vi "BuildPageArray.vi"(8 "error in (no error)":errorcluster, 10 "Config File Path":path) -> (0 "error out":errorcluster, 2 "Num Pages":i32, 3 "Array":refnum<class "Slide.lvclass">[](array[class]))   [LabVIEW 2017]
uses:
  Slide/Slide.lvclass
  Slide/SlideType.ctl
  <vilib>/regexp/Match Regular Expression.xnode
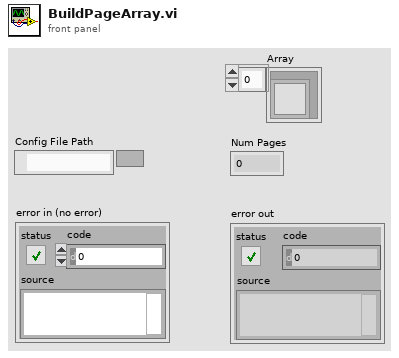
[diagram p1: front panel]
types:
  T1 = typedef "Slide.lvclass/SlideType.ctl" = enum16{"Image", "FP", "BD"}
  T2 = cluster{i32, "BD Slide":refnum<class "Slide.lvclass">}
  T3 = cluster{i32, "BD Slide":refnum<class "Slide.lvclass">}[]
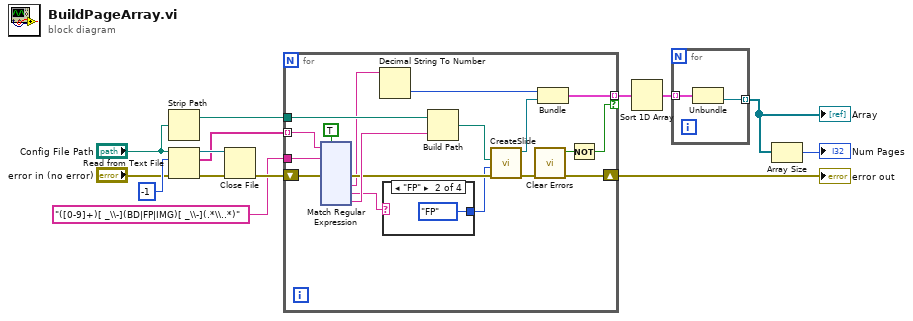
[diagram p0: block diagram]
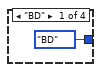
[diagram p2: hidden frame]
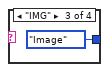
[diagram p3: hidden frame]
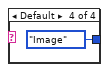
[diagram p4: hidden frame]
diagram:
  n1 = Strip Path(path="Config File Path") -> (stripped path=w6:path)  [unwired: 1 out]
  n2 = Read from Text File(file (use dialog)="Config File Path", count=-1, error in="error in (no error)") -> (refnum out=w11:refnum<file>, text=w10:string[], error out=w12:errorcluster)  [unwired: 1 in, 1 out]
  n3 = Close File(refnum=w11, error in=w12) -> (error out=w9:errorcluster)  [unwired: 1 out]
  n4 = for {
    tunnel: w10 -> [w31] mode=indexing
    shift-right: [w17] -> w4
    shift-left: w9 -> [w29]
    tunnel: "([0-9]+)[ _\\-](BD|FP|IMG)[ _\\-](.*\\..*)" -> [w28]
    tunnel: w6 -> [w27]
    tunnel: [w18] -> w3 mode=indexing if=w15
    n5 = xnode "Match Regular Expression"("input string"=w31, "regular expression"=w28, "error in"=w29, "ignore case? (F)"=TRUE) -> ("error out"=w25:errorcluster, "submatch 1"=w21:string, "submatch 2"=w26:string, "submatch 3"=w32:string)  [unwired: 2 in, 4 out]
    n6 = Decimal String To Number(string=w21) -> (number=w20:i32)  [unwired: 2 in, 1 out]
    n7 = case shown="\"FP\"" w26 {
      tunnel: [SlideType."BD" ("Type") SlideType."FP" ("Type") SlideType."Image" ("Type") SlideType."Image" ("Type")] -> w23
      frame "BD" {
      }
      frame "FP" {
      }
      frame "IMG" {
      }
      frame Default {
      }
    }
    n8 = Build Path(base path=w27, name or relative path=w32) -> (appended path=w22:path)
    n9 = call "CreateSlide.vi"("error in (no error)"=w25, "Type (FP)"=w23, "Path"=w22) -> ("error out"=w24:errorcluster, "BD Slide"=w19:refnum<class "Slide.lvclass">)  [unwired: 7 in]
    n10 = call <vilib>:"Clear Errors.vi"("error in (no error)"=w24) -> ("error out"=w17:errorcluster, "specific error cleared?"=w16:bool)  [unwired: 5 in]
    n11 = Bundle(w20, "BD Slide"=w19) -> (w18:T2)  [unwired: 1 in]
    n12 = Not(x=w16) -> (.not. x?=w15:bool)
  }
  "error out" <- w4
  n13 = Sort 1D Array(array=w3) -> (sorted array=w2:T3)
  n14 = for {
    tunnel: w2 -> [w156] mode=indexing
    tunnel: [w155] -> w1 mode=indexing
    n15 = Unbundle(w156) -> ("BD Slide"=w155:refnum<class "Slide.lvclass">)  [unwired: 1 out]
  }
  "Array" <- w1
  n16 = Array Size(array=w1) -> (size(s)=→"Num Pages":i32)
